vi "Example Enumerate - EnumerateCallback Callback.vi"(4 "EnumerateCallback":refnum<user-event>, 5 "Event Data":T1, 6 "Control Ref":refnum<k24>, 7 "Event Common Data":T2) -> ()   [LabVIEW 2013]
uses:
  C:/tf/play/labview/Tinkerforge.dll
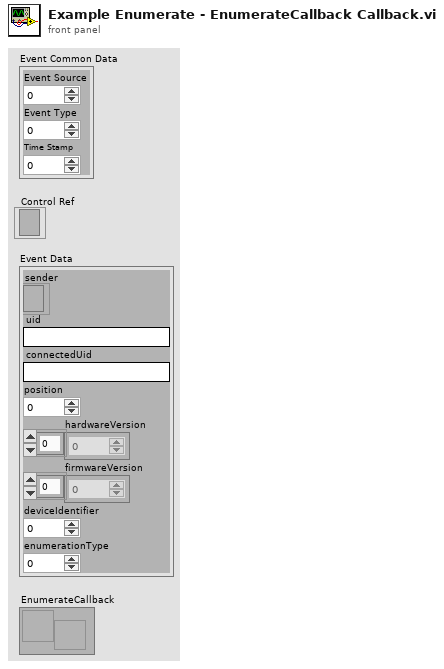
[diagram p1: front panel]
types:
  T1 = cluster{"sender":refnum<k24>, "uid":string, "connectedUid":string, "position":u16, "hardwareVersion":i16[], "firmwareVersion":i16[], "deviceIdentifier":i32, "enumerationType":i16}
  T2 = cluster{"Event Source":i32, "Event Type":u32, "Time Stamp":u32}
  T3 = cluster{"uid":string, "connectedUid":string, "position":u16, "hardwareVersion":i16[], "firmwareVersion":i16[], "deviceIdentifier":i32, "enumerationType":i16}
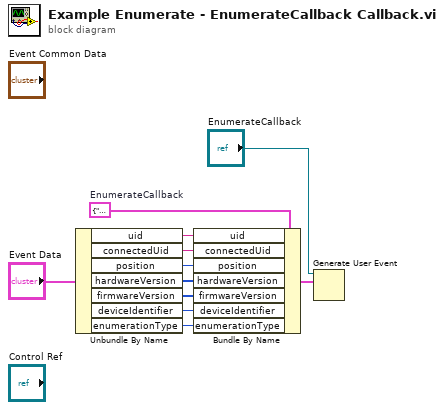
[diagram p0: block diagram]
diagram:
  w8 = T3 {"uid"="", "connectedUid"="", "position"=0, "hardwareVersion"=[], "firmwareVersion"=[], "deviceIdentifier"=0, "enumerationType"=0}  # EnumerateCallback
  n1 = Unbundle By Name("Event Data") -> ("uid"=w7:string, "connectedUid"=w6:string, "position"=w5:u16, "hardwareVersion"=w4:i16[], "firmwareVersion"=w3:i16[], "deviceIdentifier"=w2:i32, "enumerationType"=w1:i16)
  n2 = Bundle By Name(cluster=w8, "uid"=w7, "connectedUid"=w6, "position"=w5, "hardwareVersion"=w4, "firmwareVersion"=w3, "deviceIdentifier"=w2, "enumerationType"=w1) -> (w11:T3)
  n3 = Generate User Event(user event="EnumerateCallback", event data cluster=w11) -> ()  [unwired: 2 in, 2 out]
